vi "Format_Hex_String_for_File_IO.vi"(1 "Hex String in":string) -> (0 "Hex String out":string)   [LabVIEW 2019]
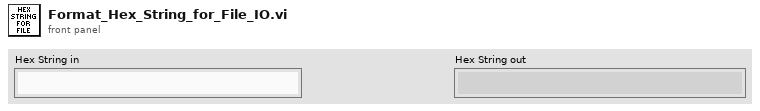
[diagram p1: front panel]
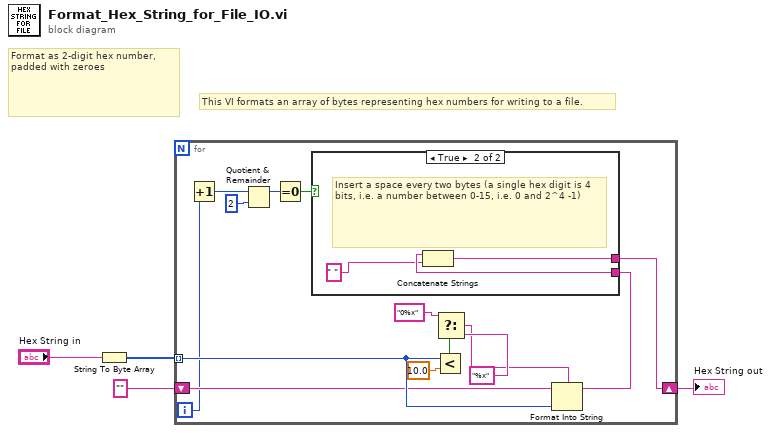
[diagram p0: block diagram]
diagram:
  # "Format as 2-digit hex number, padded with zeroes"
  # "This VI formats an array of bytes representing hex numbers for writing to a file."
  n1 = String To Byte Array(string="Hex String in") -> (unsigned byte array=w3:u8[])
  n2 = for {
    tunnel: w3 -> [w13] mode=indexing
    shift-right: [w5] -> w1
    shift-left: "" -> [w12]
    i -> [w7]
    n3 = Increment(x=w7) -> (x+1=w8:i32)
    n4 = Quotient & Remainder(x=w8, y=2) -> (x-y*floor(x/y)=w11:i32)  [unwired: 1 out]
    n5 = Equal To 0?(x=w11) -> (x = 0?=w10:bool)
    n6 = Less?(x=w13, y=10.0) -> (x < y?=w17:bool)
    n7 = Select(t="0%x", s=w17, f="%x") -> (s? t:f=w14:string)
    n8 = Format Into String(format string=w14, initial string=w12, w13) -> (resulting string=w6:string)  [unwired: 1 in, 1 out]
    n9 = case shown="True" w10 {
      tunnel: w6 -> [w19 w22]
      tunnel: [w19 w20] -> w5
      frame False {
      }
      frame True {
        # "Insert a space every two bytes (a single hex digit is 4 bits, i.e. a number between 0-15, i.e. 0 and 2^4 -1)"
        n10 = Concatenate Strings(w22, " ") -> (w20:string)
      }
    }
  }
  "Hex String out" <- w1
